vi "data_picker.vi"(8 "index":i32, 10 "Indicies":i32[](array[numeric]), 11 "Data in":T1[](array[typedef])) -> (3 "Data Out":T1)   [LabVIEW 2017]
uses:
  Box/Annular Flow/Jason/LabVIEW 2017/Input Channel Lists/analog_data.ctl
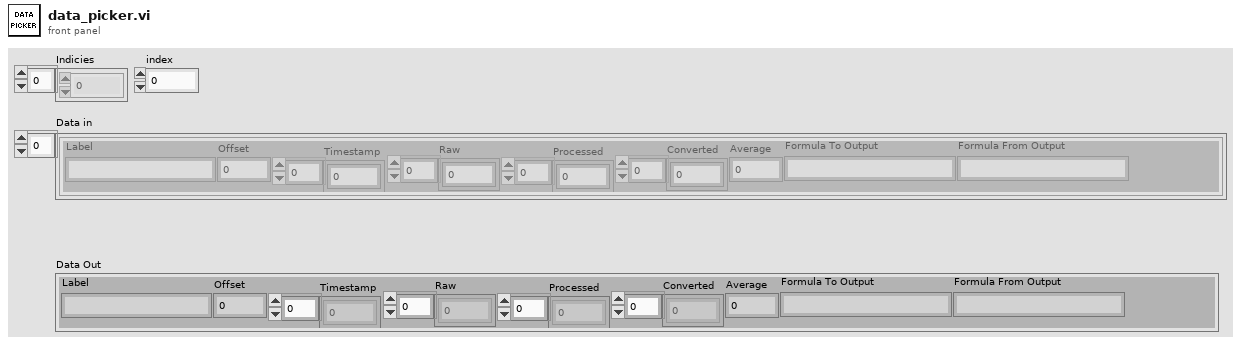
[diagram p1: front panel]
types:
  T1 = typedef "analog_data.ctl" = cluster{"Label":string, "Offset":dbl, "Timestamp":dbl[], "Raw":dbl[], "Processed":dbl[], "Converted":dbl[], "Average":dbl, "Formula To Output":string, "Formula From Output":string}
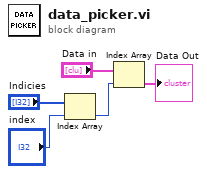
[diagram p0: block diagram]
diagram:
  n1 = Index Array(array="Indicies", index="index") -> (element=w4:i32)
  n2 = Index Array(array="Data in", index=w4) -> (element=→"Data Out":T1)
